vi "Multiple Registration - Wrong.vi"() -> ()   [LabVIEW 2011]
panel:
  out "Time Process 3 was Stopped":timestamp
  out "Process 3":timestamp
  out "Time Process 2 was Stopped":timestamp
  out "Process 2":timestamp
  out "Time Process 1 was Stopped":timestamp
  in  "stop":bool
  out "Process 1":timestamp
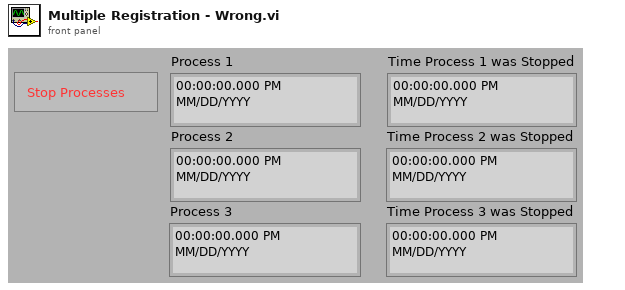
[diagram p1: front panel]
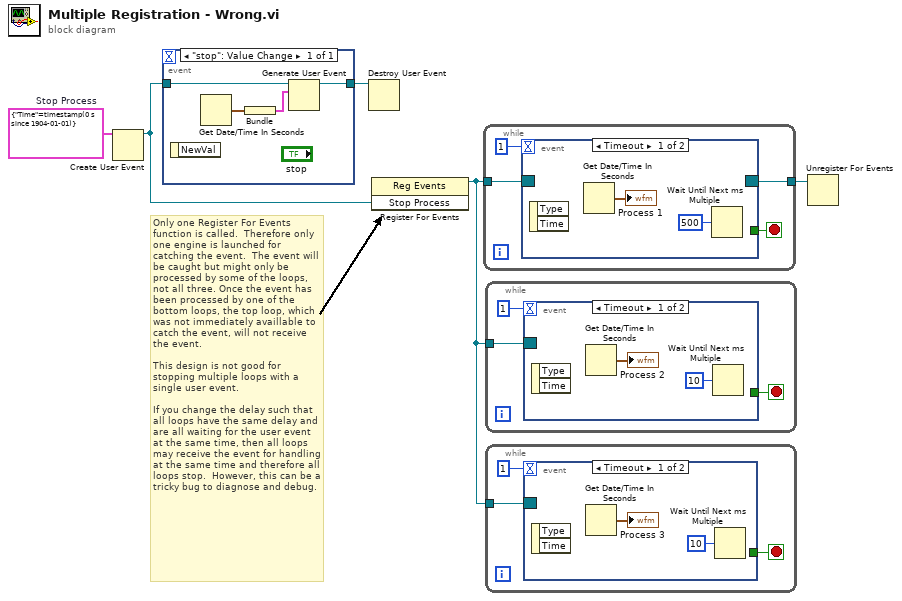
[diagram p0: block diagram]
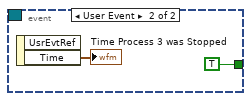
[diagram p2: hidden frame]
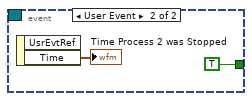
[diagram p3: hidden frame]
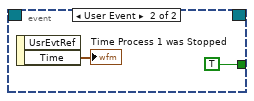
[diagram p4: hidden frame]
diagram:
  w5 = cluster{"Time":timestamp} {"Time"=timestamp(0 s since 1904-01-01)}  # Stop Process
  # "Only one Register For Events function is called.  Therefore only one engine is launched for catching the event.  The event will be caught but might only be processed by some of the loops, not all three. Once the event has been processed by one of the bottom loops, the top loop, which was not immediately availlable to catch the event, will not receive the event.\n\nThis design is not good for stopping multiple loops with a single user event.\n\nIf you change the delay such that all loops have the same delay and are all waiting for the user event at the same time, then all loops may receive the event for handling at the same time and therefore all loops stop.  However, this can be a tricky bug to diagnose and debug."
  n1 = Create User Event(user event datatype=w5) -> (user event=w4:refnum<user-event>)  [unwired: 1 in, 1 out]
  n2 = event shown="[0] \"stop\": Value Change" {
    selector: _ -> [_]
    dyn-events: _ -> [_]
    timeout: _ -> [_]
    tunnel: w4 -> [w9]
    tunnel: [w6] -> w2
    event "stop": Value Change {
      n3 = event-data() -> ()  [unwired: 1 in, 1 out]
      n4 = Get Date/Time In Seconds() -> (seconds since 1Jan1904=w8:timestamp)
      n5 = Bundle("seconds since 1Jan1904"=w8) -> (w7:cluster{"seconds since 1Jan1904":timestamp})  [unwired: 1 in]
      n6 = Generate User Event(user event=w9, event data cluster=w7) -> (user event out=w6:refnum<user-event>)  [unwired: 1 in, 1 out]
    }
  }
  n7 = Destroy User Event(user event=w2) -> ()  [unwired: 1 in, 1 out]
  n8 = register-events(w4) -> (reference out=w3:refnum<event-registration>)  [unwired: 2 in, 1 out]
  n9 = while {
    tunnel: w3 -> [w12]
    tunnel: [w10] -> w1
    stop <- w11 stop-if-true
    n10 = event shown="[0] Timeout" {
      selector: w12 -> [_ _]
      dyn-events: [_ _] -> w10
      timeout: 1 -> [_ _]
      tunnel: [_ TRUE] -> w11
      event Timeout {
        n11 = event-data() -> ()  [unwired: 1 in, 2 out]
        n12 = Get Date/Time In Seconds() -> (seconds since 1Jan1904=→"Process 1":timestamp)
        n13 = Wait Until Next ms Multiple(millisecond multiple=u32 500) -> ()  [unwired: 1 out]
      }
      event User Event {
        n14 = event-data() -> ("Time"=→"Time Process 1 was Stopped":timestamp)  [unwired: 1 in, 1 out]
      }
    }
  }
  n15 = while {
    tunnel: w3 -> [w19]
    stop <- w18 stop-if-true
    n16 = event shown="[0] Timeout" {
      selector: w19 -> [_ _]
      dyn-events: _ -> [_ _]
      timeout: 1 -> [_ _]
      tunnel: [_ TRUE] -> w18
      event Timeout {
        n17 = event-data() -> ()  [unwired: 1 in, 2 out]
        n18 = Get Date/Time In Seconds() -> (seconds since 1Jan1904=→"Process 2":timestamp)
        n19 = Wait Until Next ms Multiple(millisecond multiple=u32 10) -> ()  [unwired: 1 out]
      }
      event User Event {
        n20 = event-data() -> ("Time"=→"Time Process 2 was Stopped":timestamp)  [unwired: 1 in, 1 out]
      }
    }
  }
  n21 = while {
    tunnel: w3 -> [w26]
    stop <- w25 stop-if-true
    n22 = event shown="[0] Timeout" {
      selector: w26 -> [_ _]
      dyn-events: _ -> [_ _]
      timeout: 1 -> [_ _]
      tunnel: [_ TRUE] -> w25
      event Timeout {
        n23 = event-data() -> ()  [unwired: 1 in, 2 out]
        n24 = Get Date/Time In Seconds() -> (seconds since 1Jan1904=→"Process 3":timestamp)
        n25 = Wait Until Next ms Multiple(millisecond multiple=u32 10) -> ()  [unwired: 1 out]
      }
      event User Event {
        n26 = event-data() -> ("Time"=→"Time Process 3 was Stopped":timestamp)  [unwired: 1 in, 1 out]
      }
    }
  }
  n27 = Unregister For Events(event registration refnum=w1) -> ()  [unwired: 1 in, 1 out]
